vi "Close.vi"(8 "error in (no error)":errorcluster, 11 "Nav6DevRef":T1) -> (0 "error out":errorcluster)   [LabVIEW 2013, in "Nav6.lvlib"]
doc: "Close the Nav6 reference. This should be placed in Finish in the FRC Framework."
uses:
  Nav6.lvlib
  Nav6DevRef.ctl
  <vilib>/Rock Robotics/WPI/SerialPort/WPI_SerialPortRef.ctl
  Nav6Mode.ctl
  StopGlobal.vi
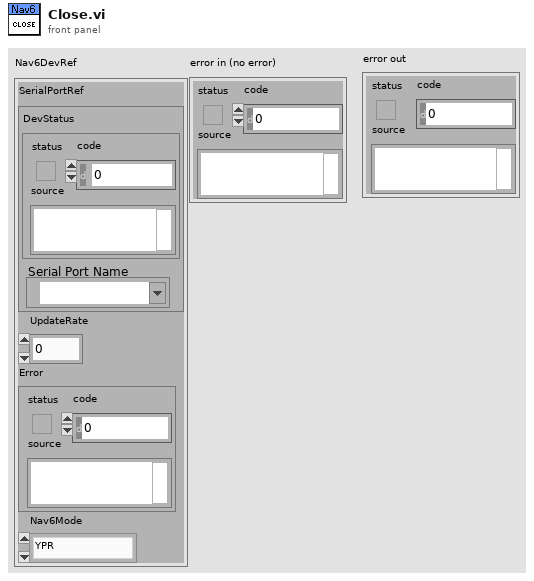
[diagram p1: front panel]
types:
  T1 = typedef "Nav6.lvlib/Nav6DevRef.ctl" = cluster{"SerialPortRef":T2, "UpdateRate":u8, "Error":errorcluster, "Nav6Mode":T3}
  T2 = typedef "WPI_SerialPortRef.ctl" = cluster{"DevStatus":errorcluster, "Serial Port Name":refnum<visa-resource-name>}
  T3 = typedef "Nav6.lvlib/Nav6Mode.ctl" = enum16{"YPR", "Gyro", "Quaternion"}
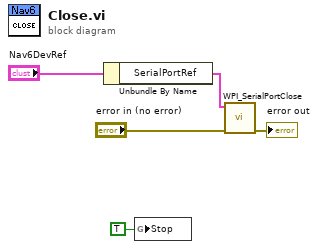
[diagram p0: block diagram]
diagram:
  n1 = Unbundle By Name("Nav6DevRef") -> ("SerialPortRef"=w4:T2)
  n2 = global write "StopGlobal.vi" "Stop"(TRUE ("Stop")) -> ()
  n3 = call <vilib>:"WPI_SerialPortClose.vi"("error in (no error)"="error in (no error)", "SerialPortRef"=w4) -> ("error out"=→"error out":errorcluster)  [unwired: 9 in]
